vi "rsscope_core_global.vi"() -> ()   [LabVIEW 2018] (continued)
"Read Callback"="", "Write Callback"="", "Supported Models"="RTO|RTP", "Instrument Options"="", "Flags"=0, "Help"="Sets the wire on which the bus signal is measured.\n\nAvailable Repeated Capabilities:\nSerialBus: SB1, SB2, SB3, SB4\r\n\nRemote-control command(s):\nBUS<m>:ARINc:POLarity"}, {"Level"=3, "Class Only"=FALSE, "Identifier"="RSSCOPE_ATTR_PROTOCOL_ARINC429_BIT_RATE_MODE", "Descriptive Name"="Protocol ARINC429 Bit Rate Mode", "Data Type"=0, "Command"="BUS{SerialBus}:ARIN:BRM", "Access"=2, "Range Table"="rsscope_rngProtocolARINC429BitRateMode", "Read Callback"="", "Write Callback"="", "Supported Models"="RTO|RTP", "Instrument Options"="", "Flags"=0, "Help"="Sets the bit rate mode to high or low speed.\n\nAvailable Repeated Capabilities:\nSerialBus: SB1, SB2, SB3, SB4\r\n\nRemote-control command(s):\nBUS<m>:ARINc:BRMode"}, {"Level"=3, "Class Only"=FALSE, "Identifier"="RSSCOPE_ATTR_PROTOCOL_ARINC429_BIT_RATE", "Descriptive Name"="Protocol ARINC429 Bit Rate", "Data Type"=0, "Command"="BUS{SerialBus}:ARIN:BRV", "Access"=2, "Range Table"="rsscope_rngProtocolARINC429BitRate", "Read Callback"="", "Write Callback"="", "Supported Models"="RTO|RTP", "Instrument Options"="", "Flags"=0, "Help"="Sets the number of transmitted bits per second.\n\nAvailable Repeated Capabilities:\nSerialBus: SB1, SB2, SB3, SB4\r\n\nRemote-control command(s):\nBUS<m>:ARINc:BRValue"}, {"Level"=3, "Class Only"=FALSE, "Identifier"="RSSCOPE_ATTR_PROTOCOL_ARINC429_THRESHOLD_HIGH", "Descriptive Name"="Protocol ARINC429 Threshold High", "Data Type"=1, "Command"="BUS{SerialBus}:ARIN:THR:HIGH", "Access"=2, "Range Table"="rsscope_rngProtocolARINC429ThresholdHigh", "Read Callback"="", "Write Callback"="", "Supported Models"="RTO|RTP", "Instrument Options"="", "Flags"=0, "Help"="Sets the high threshold level of the signal.\n\nAvailable Repeated Capabilities:\nSerialBus: SB1, SB2, SB3, SB4\r\n\nRemote-control command(s):\nBUS<m>:ARINc:THReshold:HIGH"}, {"Level"=3, "Class Only"=FALSE, "Identifier"="RSSCOPE_ATTR_PROTOCOL_ARINC429_THRESHOLD_LOW", "Descriptive Name"="Protocol ARINC429 Threshold Low", "Data Type"=1, "Command"="BUS{SerialBus}:ARIN:THR:LOW", "Access"=2, "Range Table"="rsscope_rngProtocolARINC429ThresholdLow", "Read Callback"="", "Write Callback"="", "Supported Models"="RTO|RTP", "Instrument Options"="", "Flags"=0, "Help"="Sets the low threshold level of the signal.\n\nAvailable Repeated Capabilities:\nSerialBus: SB1, SB2, SB3, SB4\r\n\nRemote-control command(s):\nBUS<m>:ARINc:THReshold:LOW"}, {"Level"=3, "Class Only"=FALSE, "Identifier"="RSSCOPE_ATTR_PROTOCOL_ARINC429_THRESHOLD_PRESET", "Descriptive Name"="Protocol ARINC429 Threshold Preset", "Data Type"=0, "Command"="BUS{SerialBus}:ARIN:PRES", "Access"=2, "Range Table"="rsscope_rngProtocolARINC429ThresholdPreset", "Read Callback"="", "Write Callback"="", "Supported Models"="RTO|RTP", "Instrument Options"="", "Flags"=0, "Help"="Sets the default threshold voltage.\n\nAvailable Repeated Capabilities:\nSerialBus: SB1, SB2, SB3, SB4\r\n\nRemote-control command(s):\nBUS<m>:ARINc:PRESet"}, {"Level"=3, "Class Only"=TRUE, "Identifier"="", "Descriptive Name"="Timing", "Data Type"=0, "Command"="", "Access"=0, "Range Table"="", "Read Callback"="", "Write Callback"="", "Supported Models"="", "Instrument Options"="", "Flags"=0, "Help"="Specifies the ranges of the timeouts."}, {"Level"=4, "Class Only"=FALSE, "Identifier"="RSSCOPE_ATTR_PROTOCOL_ARINC429_MIN_GAP_ENABLED", "Descriptive Name"="Protocol ARINC429 Min Gap Enabled", "Data Type"=3, "Command"="BUS{SerialBus}:ARIN:MING:SEL", "Access"=2, "Range Table"="", "Read Callback"="", "Write Callback"="", "Supported Models"="RTO|RTP", "Instrument Options"="", "Flags"=0, "Help"="Enables the selection of the min gap.\n\nAvailable Repeated Capabilities:\nSerialBus: SB1, SB2, SB3, SB4\r\n\nRemote-control command(s):\nBUS<m>:ARINc:MINGap:SELect"}, {"Level"=4, "Class Only"=FALSE, "Identifier"="RSSCOPE_ATTR_PROTOCOL_ARINC429_MIN_GAP_BITS", "Descriptive Name"="Protocol ARINC429 Min Gap Bits", "Data Type"=0, "Command"="BUS{SerialBus}:ARIN:MING:BITS", "Access"=2, "Range Table"="rsscope_rngProtocolARINC429MinGapBits", "Read Callback"="", "Write Callback"="", "Supported Models"="RTO|RTP", "Instrument Options"="", "Flags"=0, "Help"="Sets a value for the min timing gap between two words.\n\nAvailable Repeated Capabilities:\nSerialBus: SB1, SB2, SB3, SB4\r\n\nRemote-control command(s):\nBUS<m>:ARINc:MINGap:BITS"}, {"Level"=4, "Class Only"=FALSE, "Identifier"="RSSCOPE_ATTR_PROTOCOL_ARINC429_MAX_GAP_ENABLED", "Descriptive Name"="Protocol ARINC429 Max Gap Enabled", "Data Type"=3, "Command"="BUS{SerialBus}:ARIN:MAXG:SEL", "Access"=2, "Range Table"="", "Read Callback"="", "Write Callback"="", "Supported Models"="RTO|RTP", "Instrument Options"="", "Flags"=0, "Help"="Enables the selection of the max gap.\n\nAvailable Repeated Capabilities:\nSerialBus: SB1, SB2, SB3, SB4\r\n\nRemote-control command(s):\nBUS<m>:ARINc:MAXGap:SELect"}, {"Level"=4, "Class Only"=FALSE, "Identifier"="RSSCOPE_ATTR_PROTOCOL_ARINC429_MAX_GAP_BITS", "Descriptive Name"="Protocol ARINC429 Max Gap Bits", "Data Type"=0, "Command"="BUS{SerialBus}:ARIN:MAXG:BITS", "Access"=2, "Range Table"="rsscope_rngProtocolARINC429MaxGapBits", "Read Callback"="", "Write Callback"="", "Supported Models"="RTO|RTP", "Instrument Options"="", "Flags"=0, "Help"="Sets the value for the maximum response time.\n\nAvailable Repeated Capabilities:\nSerialBus: SB1, SB2, SB3, SB4\r\n\nRemote-control command(s):\nBUS<m>:ARINc:MAXGap:BITS"}, {"Level"=3, "Class Only"=TRUE, "Identifier"="", "Descriptive Name"="Decoding Results", "Data Type"=0, "Command"="", "Access"=0, "Range Table"="", "Read Callback"="", "Write Callback"="", "Supported Models"="", "Instrument Options"="", "Flags"=0, "Help"="Returns the decoding result of the specified word."}, {"Level"=4, "Class Only"=FALSE, "Identifier"="RSSCOPE_ATTR_PROTOCOL_ARINC429_DECODING_RESULTS_WORDS_COUNT", "Descriptive Name"="Protocol ARINC429 Decoding Results Words Count", "Data Type"=0, "Command"="BUS{SerialBus}:ARIN:WCO?", "Access"=0, "Range Table"="", "Read Callback"="", "Write Callback"="", "Supported Models"="RTO|RTP", "Instrument Options"="", "Flags"=0, "Help"="Returns the number of decoded words.\n\nAvailable Repeated Capabilities:\nSerialBus: SB1, SB2, SB3, SB4\r\n\nRemote-control command(s):\nBUS<m>:ARINc:WCOunt?"}, {"Level"=2, "Class Only"=TRUE, "Identifier"="", "Descriptive Name"="RFFE", "Data Type"=0, "Command"="", "Access"=0, "Range Table"="", "Read Callback"="", "Write Callback"="", "Supported Models"="", "Instrument Options"="", "Flags"=0, "Help"="This class contains attributes that configure the RFFE (Radio Frequency Front-End)\n\nAttributes in this class require option R&S RTO-K40."}, {"Level"=3, "Class Only"=FALSE, "Identifier"="RSSCOPE_ATTR_PROTOCOL_RFFE_CLOCK_SOURCE", "Descriptive Name"="Protocol RFFE Clock Source", "Data Type"=0, "Command"="BUS{SerialBus}:RFFE:CLOC:SOUR", "Access"=2, "Range Table"="rsscope_rngProtocolWaveformSource", "Read Callback"="", "Write Callback"="", "Supported Models"="", "Instrument Options"="K40", "Flags"=0, "Help"="Sets the source of the RFFE clock line.\n\nAvailable Repeated Capabilities:\nSerialBus: SB1, SB2, SB3, SB4\r\n\nRemote-control command(s):\nBUS<m>:RFFE:CLOCk:SOURce"}, {"Level"=3, "Class Only"=FALSE, "Identifier"="RSSCOPE_ATTR_PROTOCOL_RFFE_DATA_SOURCE", "Descriptive Name"="Protocol RFFE Data Source", "Data Type"=0, "Command"="BUS{SerialBus}:RFFE:DATA:SOUR", "Access"=2, "Range Table"="rsscope_rngProtocolWaveformSource", "Read Callback"="", "Write Callback"="", "Supported Models"="", "Instrument Options"="K40", "Flags"=0, "Help"="Sets the source of the RFFE data line.\n\nAvailable Repeated Capabilities:\nSerialBus: SB1, SB2, SB3, SB4\r\n\nRemote-control command(s):\nBUS<m>:RFFE:DATA:SOURce"}, {"Level"=3, "Class Only"=FALSE, "Identifier"="RSSCOPE_ATTR_PROTOCOL_RFFE_PRESET_THRESHOLD", "Descriptive Name"="Protocol RFFE Preset Threshold", "Data Type"=0, "Command"="BUS{SerialBus}:RFFE:PRES", "Access"=2, "Range Table"="rsscope_rngProtocolRFFEPreset", "Read Callback"="", "Write Callback"="", "Supported Models"="", "Instrument Options"="K40", "Flags"=0, "Help"="Sets default threshold voltages for 1.2 V or 1.8 V bus. Set the value to Manual if you want to define individual thresholds.\n\nAvailable Repeated Capabilities:\nSerialBus: SB1, SB2, SB3, SB4\r\n\nRemote-control command(s):\nBUS<m>:RFFE:PRESet"}, {"Level"=3, "Class Only"=FALSE, "Identifier"="RSSCOPE_ATTR_PROTOCOL_RFFE_CLOCK_THRESHOLD_HIGH", "Descriptive Name"="Protocol RFFE Clock Threshold High", "Data Type"=1, "Command"="BUS{SerialBus}:RFFE:CLOC:THR:HIGH", "Access"=2, "Range Table"="RsScope_rngProtocolRFFEThreshold", "Read Callback"="", "Write Callback"="", "Supported Models"="", "Instrument Options"="K40", "Flags"=0, "Help"="Set the positive going thresholds.\n\nAvailable Repeated Capabilities:\nSerialBus: SB1, SB2, SB3, SB4\r\n\nRemote-control command(s):\nBUS<m>:RFFE:CLOCk:THReshold:HIGH"}, {"Level"=3, "Class Only"=FALSE, "Identifier"="RSSCOPE_ATTR_PROTOCOL_RFFE_CLOCK_THRESHOLD_LOW", "Descriptive Name"="Protocol RFFE Clock Threshold Low", "Data Type"=1, "Command"="BUS{SerialBus}:RFFE:CLOC:THR:LOW", "Access"=2, "Range Table"="RsScope_rngProtocolRFFEThreshold", "Read Callback"="", "Write Callback"="", "Supported Models"="", "Instrument Options"="K40", "Flags"=0, "Help"="Sets the negative going thresholds.\n\nAvailable Repeated Capabilities:\nSerialBus: SB1, SB2, SB3, SB4\r\n\nRemote-control command(s):\nBUS<m>:RFFE:CLOCk:THReshold:LOW"}, {"Level"=3, "Class Only"=FALSE, "Identifier"="RSSCOPE_ATTR_PROTOCOL_RFFE_CLOCK_THRESHOLD_HYSTERESIS", "Descriptive Name"="Protocol RFFE Clock Threshold Hysteresis", "Data Type"=1, "Command"="BUS{SerialBus}:RFFE:CLOC:THR:HYST", "Access"=2, "Range Table"="rsscope_rngProtocolRFFEThresholdHysteresis", "Read Callback"="", "Write Callback"="", "Supported Models"="", "Instrument Options"="K40", "Flags"=0, "Help"="Sets the hysteresises between V TP  and V TN.\n\nAvailable Repeated Capabilities:\nSerialBus: SB1, SB2, SB3, SB4\r\n\nRemote-control command(s):\nBUS<m>:RFFE:CLOCk:THReshold:HYSTeresis"}, {"Level"=3, "Class Only"=FALSE, "Identifier"="RSSCOPE_ATTR_PROTOCOL_RFFE_DATA_THRESHOLD_HIGH", "Descriptive Name"="Protocol RFFE Data Threshold High", "Data Type"=1, "Command"="BUS{SerialBus}:RFFE:DATA:THR:HIGH", "Access"=2, "Range Table"="RsScope_rngProtocolRFFEThreshold", "Read Callback"="", "Write Callback"="", "Supported Models"="", "Instrument Options"="K40", "Flags"=0, "Help"="Set the positive going thresholds.\n\nAvailable Repeated Capabilities:\nSerialBus: SB1, SB2, SB3, SB4\r\n\nRemote-control command(s):\nBUS<m>:RFFE:DATA:THReshold:HIGH"}, {"Level"=3, "Class Only"=FALSE, "Identifier"="RSSCOPE_ATTR_PROTOCOL_RFFE_DATA_THRESHOLD_LOW", "Descriptive Name"="Protocol RFFE Data Threshold Low", "Data Type"=1, "Command"="BUS{SerialBus}:RFFE:DATA:THR:LOW", "Access"=2, "Range Table"="RsScope_rngProtocolRFFEThreshold", "Read Callback"="", "Write Callback"="", "Supported Models"="", "Instrument Options"="K40", "Flags"=0, "Help"="Sets the negative going thresholds.\n\nAvailable Repeated Capabilities:\nSerialBus: SB1, SB2, SB3, SB4\r\n\nRemote-control command(s):\nBUS<m>:RFFE:DATA:THReshold:LOW"}, {"Level"=3, "Class Only"=FALSE, "Identifier"="RSSCOPE_ATTR_PROTOCOL_RFFE_DATA_THRESHOLD_HYSTERESIS", "Descriptive Name"="Protocol RFFE Data Threshold Hysteresis", "Data Type"=1, "Command"="BUS{SerialBus}:RFFE:DATA:THR:HYST", "Access"=2, "Range Table"="rsscope_rngProtocolRFFEThresholdHysteresis", "Read Callback"="", "Write Callback"="", "Supported Models"="", "Instrument Options"="K40", "Flags"=0, "Help"="Sets the hysteresises between V TP  and V TN.\n\nAvailable Repeated Capabilities:\nSerialBus: SB1, SB2, SB3, SB4\r\n\nRemote-control command(s):\nBUS<m>:RFFE:DATA:THReshold:HYSTeresis"}, {"Level"=3, "Class Only"=FALSE, "Identifier"="RSSCOPE_ATTR_PROTOCOL_RFFE_THRESHOLDS_COUPLING", "Descriptive Name"="Protocol RFFE Thresholds Coupling", "Data Type"=3, "Command"="BUS{SerialBus}:RFFE:COUP", "Access"=2, "Range Table"="", "Read Callback"="", "Write Callback"="", "Supported Models"="", "Instrument Options"="K40", "Flags"=0, "Help"="If enabled, the data line thresholds are set to the clock line threshold values.\n\nAvailable Repeated Capabilities:\nSerialBus: SB1, SB2, SB3, SB4\r\n\nRemote-control command(s):\nBUS<m>:RFFE:COUPling"}, {"Level"=3, "Class Only"=FALSE, "Identifier"="RSSCOPE_ATTR_PROTOCOL_RFFE_GLITCH_FILTER_ENABLED", "Descriptive Name"="Protocol RFFE Glitch Filter Enabled", "Data Type"=3, "Command"="BUS{SerialBus}:RFFE:GFIL", "Access"=2, "Range Table"="", "Read Callback"="", "Write Callback"="", "Supported Models"="", "Instrument Options"="K40", "Flags"=0, "Help"="Enables the glitch filter on the clock and data lines to improve decode accuracy.\n\nAvailable Repeated Capabilities:\nSerialBus: SB1, SB2, SB3, SB4\r\n\nRemote-control command(s):\nBUS<m>:RFFE:GFILter"}, {"Level"=3, "Class Only"=FALSE, "Identifier"="RSSCOPE_ATTR_PROTOCOL_RFFE_GLITCH_FILTER_WIDTH", "Descriptive Name"="Protocol RFFE Glitch Filter Width", "Data Type"=1, "Command"="BUS{SerialBus}:RFFE:GFW", "Access"=2, "Range Table"="rsscope_rngProtocolRFFEGlitchFilterWidth", "Read Callback"="", "Write Callback"="", "Supported Models"="", "Instrument Options"="K40", "Flags"=0, "Help"="Sets the maximum glitch width to be ignored\n\nAvailable Repeated Capabilities:\nSerialBus: SB1, SB2, SB3, SB4\r\n\nRemote-control command(s):\nBUS<m>:RFFE:GFWidth"}, {"Level"=3, "Class Only"=FALSE, "Identifier"="RSSCOPE_ATTR_PROTOCOL_RFFE_MIN_GAP_ENABLED", "Descriptive Name"="Protocol RFFE Min Gap Enabled", "Data Type"=3, "Command"="BUS{SerialBus}:RFFE:MING:SEL", "Access"=2, "Range Table"="", "Read Callback"="", "Write Callback"="", "Supported Models"="", "Instrument Options"="K40", "Flags"=0, "Help"="Enables the selection of the min gap.\n\nAvailable Repeated Capabilities:\nSerialBus: SB1, SB2, SB3, SB4\r\n\nRemote-control command(s):\nBUS<m>:RFFE:MINGap:SELect"}, {"Level"=3, "Class Only"=FALSE, "Identifier"="RSSCOPE_ATTR_PROTOCOL_RFFE_MIN_GAP_TIME", "Descriptive Name"="Protocol RFFE Min Gap Time", "Data Type"=1, "Command"="BUS{SerialBus}:RFFE:MING:TIME", "Access"=2, "Range Table"="rsscope_rngProtocolRFFEMinGapTime", "Read Callback"="", "Write Callback"="", "Supported Models"="", "Instrument Options"="K40", "Flags"=0, "Help"="Sets the minimum idle time between the Bus Park Cycle (BP) and Sequence Start Condition (SSC).\n\nAvailable Repeated Capabilities:\nSerialBus: SB1, SB2, SB3, SB4\r\n\nRemote-control command(s):\nBUS<m>:RFFE:MINGap:TIME"}, {"Level"=3, "Class Only"=FALSE, "Identifier"="RSSCOPE_ATTR_PROTOCOL_RFFE_MAX_GAP_ENABLED", "Descriptive Name"="Protocol RFFE Max Gap Enabled", "Data Type"=3, "Command"="BUS{SerialBus}:RFFE:MAXG:SEL", "Access"=2, "Range Table"="", "Read Callback"="", "Write Callback"="", "Supported Models"="", "Instrument Options"="K40", "Flags"=0, "Help"="Enables the selection of the max gap.\n\nAvailable Repeated Capabilities:\nSerialBus: SB1, SB2, SB3, SB4\r\n\nRemote-control command(s):\nBUS<m>:RFFE:MAXGap:SELect"}, {"Level"=3, "Class Only"=FALSE, "Identifier"="RSSCOPE_ATTR_PROTOCOL_RFFE_MAX_GAP_TIME", "Descriptive Name"="Protocol RFFE Max Gap Time", "Data Type"=1, "Command"="BUS{SerialBus}:RFFE:MAXG:TIME", "Access"=2, "Range Table"="RsScope_rngProtocolRFFEMaxGapTime", "Read Callback"="", "Write Callback"="", "Supported Models"="", "Instrument Options"="K40", "Flags"=0, "Help"="Sets the maximum idle time between the Bus Park Cycle (BP) and Sequence Start Condition (SSC).\n\nAvailable Repeated Capabilities:\nSerialBus: SB1, SB2, SB3, SB4\r\n\nRemote-control command(s):\nBUS<m>:RFFE:MAXGap:TIME"}, {"Level"=3, "Class Only"=FALSE, "Identifier"="RSSCOPE_ATTR_PROTOCOL_RFFE_READ_MODE", "Descriptive Name"="Protocol RFFE Read Mode", "Data Type"=0, "Command"="BUS{SerialBus}:RFFE:RDMD", "Access"=2, "Range Table"="RsScope_rngRFFEReadMode", "Read Callback"="", "Write Callback"="", "Supported Models"="", "Instrument Options"="K40", "Flags"=0, "Help"="Selects, if the standard or synchronous read (SREAD) mode is used.\n\nAvailable Repeated Capabilities:\nSerialBus: SB1, SB2, SB3, SB4\r\n\nRemote-control command(s):\nBUS<m>:RFFE:RDMD"}, {"Level"=3, "Class Only"=FALSE, "Identifier"="RSSCOPE_ATTR_PROTOCOL_RFFE_VERSION", "Descriptive Name"="Protocol RFFE Version", "Data Type"=0, "Command"="BUS{SerialBus}:RFFE:VERS", "Access"=2, "Range Table"="RsScope_rngRFFEVersion", "Read Callback"="", "Write Callback"="", "Supported Models"="", "Instrument Options"="K40", "Flags"=0, "Help"="Selects the RFFE version.\n\nAvailable Repeated Capabilities:\nSerialBus: SB1, SB2, SB3, SB4\r\n\nRemote-control command(s):\nBUS<m>:RFFE:VERSion"}, {"Level"=3, "Class Only"=TRUE, "Identifier"="", "Descriptive Name"="Decoding Results", "Data Type"=0, "Command"="", "Access"=0, "Range Table"="", "Read Callback"="", "Write Callback"="", "Supported Models"="", "Instrument Options"="", "Flags"=0, "Help"="Returns the decoding result of the specified sequence."}, {"Level"=4, "Class Only"=FALSE, "Identifier"="RSSCOPE_ATTR_PROTOCOL_RFFE_DECODING_RESULTS_SEQUENCE_COUNT", "Descriptive Name"="Protocol RFFE Decoding Results Sequence Count", "Data Type"=0, "Command"="BUS{SerialBus}:RFFE:FCO?", "Access"=0, "Range Table"="", "Read Callback"="", "Write Callback"="", "Supported Models"="RTO|RTP", "Instrument Options"="", "Flags"=0, "Help"="Returns the number of command sequences in the current acquisition.\n\nAvailable Repeated Capabilities:\nSerialBus: SB1, SB2, SB3, SB4\r\n\nRemote-control command(s):\nBUS<m>:RFFE:FCOunt?"}, {"Level"=2, "Class Only"=TRUE, "Identifier"="", "Descriptive Name"="MDIO", "Data Type"=0, "Command"="", "Access"=0, "Range Table"="", "Read Callback"="", "Write Callback"="", "Supported Models"="", "Instrument Options"="", "Flags"=0, "Help"="This class contains attributes that configure the MDIO (Manage-\nment Data Input/Output)\n\nFunctions in this class requires option R&S RTO-K55."}, {"Level"=3, "Class Only"=FALSE, "Identifier"="RSSCOPE_ATTR_PROTOCOL_MDIO_THRESHOLD_PRESET", "Descriptive Name"="Protocol MDIO Threshold Preset", "Data Type"=0, "Command"="BUS{SerialBus}:MDIO:PRES", "Access"=2, "Range Table"="rsscope_rngProtocolMDIOThresholdPreset", "Read Callback"="", "Write Callback"="", "Supported Models"="", "Instrument Options"="K55", "Flags"=0, "Help"="Selects the default threshold settings according to the Ethernet standard.\n\nAvailable Repeated Capabilities:\nSerialBus: SB1, SB2, SB3, SB4\r\n\nRemote-control command(s):\nBUS<m>:MDIO:PRESet"}, {"Level"=3, "Class Only"=FALSE, "Identifier"="RSSCOPE_ATTR_PROTOCOL_MDIO_CLOCK_SOURCE", "Descriptive Name"="Protocol MDIO Clock Source", "Data Type"=0, "Command"="BUS{SerialBus}:MDIO:CLOC:SOUR", "Access"=2, "Range Table"="rsscope_rngProtocolWaveformSource", "Read Callback"="", "Write Callback"="", "Supported Models"="", "Instrument Options"="K55", "Flags"=0, "Help"="Selects the source for the clock line (management data clock, MDC). Permitted selections are the analog channels &apos;C1&apos;  &apos;C4&apos; and the digital channels &apos;D0&apos;  &apos;D15&apos;.\n\nAvailable Repeated Capabilities:\nSerialBus: SB1, SB2, SB3, SB4\r\n\nRemote-control command(s):\nBUS<m>:MDIO:CLOCk:SOURce"}, {"Level"=3, "Class Only"=FALSE, "Identifier"="RSSCOPE_ATTR_PROTOCOL_MDIO_CLOCK_THRESHOLD_HIGH", "Descriptive Name"="Protocol MDIO Clock Threshold High", "Data Type"=1, "Command"="BUS{SerialBus}:MDIO:CLOC:THR:HIGH", "Access"=2, "Range Table"="rsscope_rngProtocolMDIOThreshold", "Read Callback"="", "Write Callback"="", "Supported Models"="", "Instrument Options"="K55", "Flags"=0, "Help"="Defines the upper threshold level for the clock signal.\n\nAvailable Repeated Capabilities:\nSerialBus: SB1, SB2, SB3, SB4\r\n\nRemote-control command(s):\nBUS<m>:MDIO:CLOCk:THReshold:HIGH"}, {"Level"=3, "Class Only"=FALSE, "Identifier"="RSSCOPE_ATTR_PROTOCOL_MDIO_CLOCK_THRESHOLD_LOW", "Descriptive Name"="Protocol MDIO Clock Threshold Low", "Data Type"=1, "Command"="BUS{SerialBus}:MDIO:CLOC:THR:LOW", "Access"=2, "Range Table"="rsscope_rngProtocolMDIOThreshold", "Read Callback"="", "Write Callback"="", "Supported Models"="", "Instrument Options"="K55", "Flags"=0, "Help"="Defines the lower threshold level for the clock signal.\n\nAvailable Repeated Capabilities:\nSerialBus: SB1, SB2, SB3, SB4\r\n\nRemote-control command(s):\nBUS<m>:MDIO:CLOCk:THReshold:LOW"}, {"Level"=3, "Class Only"=FALSE, "Identifier"="RSSCOPE_ATTR_PROTOCOL_MDIO_DATA_SOURCE", "Descriptive Name"="Protocol MDIO Data Source", "Data Type"=0, "Command"="BUS{SerialBus}:MDIO:DATA:SOUR", "Access"=2, "Range Table"="rsscope_rngProtocolWaveformSource", "Read Callback"="", "Write Callback"="", "Supported Models"="", "Instrument Options"="K55", "Flags"=0, "Help"="Selects the source for the data signal. Permitted selections are the analog channels &apos;C1&apos;  &apos;C4&apos; and the digital channels &apos;D0&apos;  &apos;D15&apos;.\n\nAvailable Repeated Capabilities:\nSerialBus: SB1, SB2, SB3, SB4\r\n\nRemote-control command(s):\nBUS<m>:MDIO:DATA:SOURce"}, {"Level"=3, "Class Only"=FALSE, "Identifier"="RSSCOPE_ATTR_PROTOCOL_MDIO_DATA_THRESHOLD_HIGH", "Descriptive Name"="Protocol MDIO Data Threshold High", "Data Type"=1, "Command"="BUS{SerialBus}:MDIO:DATA:THR:HIGH", "Access"=2, "Range Table"="rsscope_rngProtocolMDIOThreshold", "Read Callback"="", "Write Callback"="", "Supported Models"="", "Instrument Options"="K55", "Flags"=0, "Help"="Defines the upper threshold level for the data signal.\n\nAvailable Repeated Capabilities:\nSerialBus: SB1, SB2, SB3, SB4\r\n\nRemote-control command(s):\nBUS<m>:MDIO:DATA:THReshold:HIGH"}, {"Level"=3, "Class Only"=FALSE, "Identifier"="RSSCOPE_ATTR_PROTOCOL_MDIO_DATA_THRESHOLD_LOW", "Descriptive Name"="Protocol MDIO Data Threshold Low", "Data Type"=1, "Command"="BUS{SerialBus}:MDIO:DATA:THR:LOW", "Access"=2, "Range Table"="rsscope_rngProtocolMDIOThreshold", "Read Callback"="", "Write Callback"="", "Supported Models"="", "Instrument Options"="K55", "Flags"=0, "Help"="Defines the lower threshold level for the data signal.\n\nAvailable Repeated Capabilities:\nSerialBus: SB1, SB2, SB3, SB4\r\n\nRemote-control command(s):\nBUS<m>:MDIO:DATA:THReshold:LOW"}, {"Level"=3, "Class Only"=FALSE, "Identifier"="RSSCOPE_ATTR_PROTOCOL_MDIO_THRESHOLDS_COUPLING", "Descriptive Name"="Protocol MDIO Thresholds Coupling", "Data Type"=3, "Command"="BUS{SerialBus}:MDIO:COUP", "Access"=2, "Range Table"="", "Read Callback"="", "Write Callback"="", "Supported Models"="", "Instrument Options"="K55", "Flags"=0, "Help"="If enabled, the data line thresholds are set to the clock line threshold values.\n\nAvailable Repeated Capabilities:\nSerialBus: SB1, SB2, SB3, SB4\r\n\nRemote-control command(s):\nBUS<m>:MDIO:COUPling"}, {"Level"=3, "Class Only"=FALSE, "Identifier"="RSSCOPE_ATTR_PROTOCOL_MDIO_MAX_GAP_TIME", "Descriptive Name"="Protocol MDIO Max Gap Time", "Data Type"=1, "Command"="BUS{SerialBus}:MDIO:MAXG", "Access"=2, "Range Table"="RsScope_rngMDIOMaxGapTime", "Read Callback"="", "Write Callback"="", "Supported Models"="", "Instrument Options"="", "Flags"=0, "Help"="Sets the maximum idle time between two frames.\n\nAvailable Repeated Capabilities:\nSerialBus: SB1, SB2, SB3, SB4\r\n\nRemote-control command(s):\nBUS<m>:MDIO:MAXGap"}, {"Level"=3, "Class Only"=TRUE, "Identifier"="", "Descriptive Name"="Decoding Results", "Data Type"=0, "Command"="", "Access"=0, "Range Table"="", "Read Callback"="", "Write Callback"="", "Supported Models"="", "Instrument Options"="", "Flags"=0, "Help"="Returns the decoding result of the specified word."}, {"Level"=4, "Class Only"=FALSE, "Identifier"="RSSCOPE_ATTR_PROTOCOL_MDIO_DECODING_RESULTS_WORD_COUNT", "Descriptive Name"="Protocol MDIO Decoding Results Word Count", "Data Type"=0, "Command"="BUS{SerialBus}:MDIO:WCO?", "Access"=0, "Range Table"="", "Read Callback"="", "Write Callback"="", "Supported Models"="", "Instrument Options"="K55", "Flags"=0, "Help"="Returns the number of decoded words.\n\nAvailable Repeated Capabilities:\nSerialBus: SB1, SB2, SB3, SB4\r\n\nRemote-control command(s):\nBUS<m>:MDIO:WCOunt?"}, {"Level"=2, "Class Only"=TRUE, "Identifier"="", "Descriptive Name"="Ethernet", "Data Type"=0, "Command"="", "Access"=0, "Range Table"="", "Read Callback"="", "Write Callback"="", "Supported Models"="", "Instrument Options"="", "Flags"=0, "Help"="This class contains attributes that configure the  Ethernet protocol variants 10BASE-T and 100BASE-TX.\n\nAttributes in this class require option R&S RTO-K8."}, {"Level"=3, "Class Only"=FALSE, "Identifier"="RSSCOPE_ATTR_PROTOCOL_ETHERNET_VARIANT", "Descriptive Name"="Protocol Ethernet Variant", "Data Type"=0, "Command"="BUS{SerialBus}:ETH:VAR", "Access"=2, "Range Table"="rsscope_rngProtocolEthernetVariant", "Read Callback"="", "Write Callback"="", "Supported Models"="", "Instrument Options"="K8", "Flags"=0, "Help"="Selects the Ethernet protocol variant and transmission speed.\n\nAvailable Repeated Capabilities:\nSerialBus: SB1, SB2, SB3, SB4\r\n\nRemote-control command(s):\nBUS<m>:ETHernet:VARiant"}, {"Level"=3, "Class Only"=FALSE, "Identifier"="RSSCOPE_ATTR_PROTOCOL_ETHERNET_SOURCE", "Descriptive Name"="Protocol Ethernet Source", "Data Type"=0, "Command"="BUS{SerialBus}:ETH:SOUR", "Access"=2, "Range Table"="rsscope_rngProtocolWaveformSource", "Read Callback"="", "Write Callback"="", "Supported Models"="", "Instrument Options"="K8", "Flags"=0, "Help"="Selects the source channel for the data signal. Usually, the source is one of the analog channels. Reference and math waveforms are available as source if the trigger source is one of the analog channels but not the serial\nbus.\n\nAvailable Repeated Capabilities:\nSerialBus: SB1, SB2, SB3, SB4\r\n\nRemote-control command(s):\nBUS<m>:ETHernet:SOURce"}, {"Level"=3, "Class Only"=FALSE, "Identifier"="RSSCOPE_ATTR_PROTOCOL_ETHERNET_POLARITY", "Descriptive Name"="Protocol Ethernet Polarity", "Data Type"=0, "Command"="BUS{SerialBus}:ETH:POL", "Access"=2, "Range Table"="rsscope_rngEthernetPolarity", "Read Callback"="", "Write Callback"="", "Supported Models"="", "Instrument Options"="K8", "Flags"=0, "Help"="Defines the polarity of the data signal. This setting is only available in 10BASE-T.\n\nAvailable Repeated Capabilities:\nSerialBus: SB1, SB2, SB3, SB4\r\n\nRemote-control command(s):\nBUS<m>:ETHernet:POLarity"}, {"Level"=3, "Class Only"=FALSE, "Identifier"="RSSCOPE_ATTR_PROTOCOL_ETHERNET_THRESHOLD_PRESET", "Descriptive Name"="Protocol Ethernet Threshold Preset", "Data Type"=0, "Command"="BUS{SerialBus}:ETH:PRES", "Access"=2, "Range Table"="rsscope_rngProtocolEthernetThresholdPreset", "Read Callback"="", "Write Callback"="", "Supported Models"="", "Instrument Options"="K8", "Flags"=0, "Help"="Sets the thresholds to predefined or individually definable voltage levels.\n\nAvailable Repeated Capabilities:\nSerialBus: SB1, SB2, SB3, SB4\r\n\nRemote-control command(s):\nBUS<m>:ETHernet:PRESet"}, {"Level"=3, "Class Only"=FALSE, "Identifier"="RSSCOPE_ATTR_PROTOCOL_ETHERNET_THRESHOLD_LOW", "Descriptive Name"="Protocol Ethernet Threshold Low", "Data Type"=1, "Command"="BUS{SerialBus}:ETH:THR:LOW", "Access"=2, "Range Table"="rsscope_rngProtocolEthernetThresholdLow", "Read Callback"="", "Write Callback"="", "Supported Models"="", "Instrument Options"="K8", "Flags"=0, "Help"="Sets the lower threshold value for the signal digitization. If the signal value is below this threshold, the signal state is considered low.\n\nAvailable Repeated Capabilities:\nSerialBus: SB1, SB2, SB3, SB4\r\n\nRemote-control command(s):\nBUS<m>:ETHernet:THReshold:LOW"}, {"Level"=3, "Class Only"=FALSE, "Identifier"="RSSCOPE_ATTR_PROTOCOL_ETHERNET_THRESHOLD_HIGH", "Descriptive Name"="Protocol Ethernet Threshold High", "Data Type"=1, "Command"="BUS{SerialBus}:ETH:THR:HIGH", "Access"=2, "Range Table"="rsscope_rngProtocolEthernetThresholdHigh", "Read Callback"="", "Write Callback"="", "Supported Models"="", "Instrument Options"="K8", "Flags"=0, "Help"="Sets the upper threshold value for the signal digitization. If the signal value is higher than the this threshold, the signal state is considered high.\n\nAvailable Repeated Capabilities:\nSerialBus: SB1, SB2, SB3, SB4\r\n\nRemote-control command(s):\nBUS<m>:ETHernet:THReshold:HIGH"}, {"Level"=3, "Class Only"=FALSE, "Identifier"="RSSCOPE_ATTR_PROTOCOL_ETHERNET_BIT_RATE", "Descriptive Name"="Protocol Ethernet Bit Rate", "Data Type"=0, "Command"="BUS{SerialBus}:ETH:BITR", "Access"=2, "Range Table"="rsscope_rngProtocolEthernetBitRate", "Read Callback"="", "Write Callback"="", "Supported Models"="", "Instrument Options"="K8", "Flags"=0, "Help"="Sets the bit rate value that defines the transmission speed in bits per second.\n\nAvailable Repeated Capabilities:\nSerialBus: SB1, SB2, SB3, SB4\r\n\nRemote-control command(s):\nBUS<m>:ETHernet:BITRate"}, {"Level"=3, "Class Only"=TRUE, "Identifier"="", "Descriptive Name"="Decoding Results", "Data Type"=0, "Command"="", "Access"=0, "Range Table"="", "Read Callback"="", "Write Callback"="", "Supported Models"="", "Instrument Options"="", "Flags"=0, "Help"="Returns the decoding result of the specified word."}, {"Level"=4, "Class Only"=FALSE, "Identifier"="RSSCOPE_ATTR_PROTOCOL_ETHERNET_DECODING_RESULTS_WORD_COUNT", "Descriptive Name"="Protocol Ethernet Decoding Results Word Count", "Data Type"=0, "Command"="BUS{SerialBus}:ETH:WCO?", "Access"=0, "Range Table"="", "Read Callback"="", "Write Callback"="", "Supported Models"="", "Instrument Options"="K8", "Flags"=0, "Help"="Returns the number of decoded words.\n\nAvailable Repeated Capabilities:\nSerialBus: SB1, SB2, SB3, SB4\r\n\nRemote-control command(s):\nBUS<m>:ETHernet:WCOunt?"}, {"Level"=2, "Class Only"=TRUE, "Identifier"="", "Descriptive Name"="USB", "Data Type"=0, "Command"="", "Access"=0, "Range Table"="", "Read Callback"="", "Write Callback"="", "Supported Models"="", "Instrument Options"="", "Flags"=0, "Help"="This class contains functions that configure the USB (Universal\nSerial Bus).\n\nFunctions in this class requires option R&S RTO-K60."}, {"Level"=3, "Class Only"=FALSE, "Identifier"="RSSCOPE_ATTR_PROTOCOL_USB_D_PLUS_SOURCE", "Descriptive Name"="Protocol USB D Plus Source", "Data Type"=0, "Command"="BUS{SerialBus}:USB:DPL:SOUR", "Access"=2, "Range Table"="rsscope_rngProtocolUSBWaveformSource", "Read Callback"="", "Write Callback"="", "Supported Models"="", "Instrument Options"="K60", "Flags"=0, "Help"="Selects the source for the D+ data signal (in USB low speed and USB full speed protocol, only).\n\nAvailable Repeated Capabilities:\nSerialBus: SB1, SB2, SB3, SB4\r\n\nRemote-control command(s):\nBUS<m>:USB:DPLus:SOURce"}, {"Level"=3, "Class Only"=FALSE, "Identifier"="RSSCOPE_ATTR_PROTOCOL_USB_D_MINUS_SOURCE", "Descriptive Name"="Protocol USB D Minus Source", "Data Type"=0, "Command"="BUS{SerialBus}:USB:DMIN:SOUR", "Access"=2, "Range Table"="rsscope_rngProtocolUSBWaveformSource", "Read Callback"="", "Write Callback"="", "Supported Models"="", "Instrument Options"="K60", "Flags"=0, "Help"="Selects the source for the D- data signal (in USB low speed and USB full speed protocol, only).\n\nAvailable Repeated Capabilities:\nSerialBus: SB1, SB2, SB3, SB4\r\n\nRemote-control command(s):\nBUS<m>:USB:DMINus:SOURce"}, {"Level"=3, "Class Only"=FALSE, "Identifier"="RSSCOPE_ATTR_PROTOCOL_USB_DIFFERENTIAL_SOURCE", "Descriptive Name"="Protocol USB Differential Source", "Data Type"=0, "Command"="BUS{SerialBus}:USB:DIFF:SOUR", "Access"=2, "Range Table"="rsscope_rngProtocolUSBWaveformSource", "Read Callback"="", "Write Callback"="", "Supported Models"="", "Instrument Options"="K60", "Flags"=0, "Help"="Selects the source for the differential signal in the USB high speed protocol.\n\nAvailable Repeated Capabilities:\nSerialBus: SB1, SB2, SB3, SB4\r\n\nRemote-control command(s):\nBUS<m>:USB:DIFFerential:SOURce"}, {"Level"=3, "Class Only"=FALSE, "Identifier"="RSSCOPE_ATTR_PROTOCOL_USB_DATA_SOURCE", "Descriptive Name"="Protocol USB Data Source", "Data Type"=0, "Command"="BUS{SerialBus}:USB:DATA:SOUR", "Access"=2, "Range Table"="rsscope_rngProtocolUSBWaveformSource", "Read Callback"="", "Write Callback"="", "Supported Models"="", "Instrument Options"="K60", "Flags"=0, "Help"="Selects the source for the data signal in the USB HSIC protocol.\n\nAvailable Repeated Capabilities:\nSerialBus: SB1, SB2, SB3, SB4\r\n\nRemote-control command(s):\nBUS<m>:USB:DATA:SOURce"}, {"Level"=3, "Class Only"=FALSE, "Identifier"="RSSCOPE_ATTR_PROTOCOL_USB_STROBE_SOURCE", "Descriptive Name"="Protocol USB Strobe Source", "Data Type"=0, "Command"="BUS{SerialBus}:USB:STR:SOUR", "Access"=2, "Range Table"="rsscope_rngProtocolUSBWaveformSource", "Read Callback"="", "Write Callback"="", "Supported Models"="", "Instrument Options"="K60", "Flags"=0, "Help"="Selects the source for the strobe signal in the USB HSIC protocol.\n\nAvailable Repeated Capabilities:\nSerialBus: SB1, SB2, SB3, SB4\r\n\nRemote-control command(s):\nBUS<m>:USB:STRobe:SOURce"}, {"Level"=3, "Class Only"=FALSE, "Identifier"="RSSCOPE_ATTR_PROTOCOL_USB_TECHNOLOGY", "Descriptive Name"="Protocol USB Technology", "Data Type"=0, "Command"="BUS{SerialBus}:USB:TECH", "Access"=2, "Range Table"="rsscope_rngProtocolUSBTechnology", "Read Callback"="", "Write Callback"="", "Supported Models"="", "Instrument Options"="K60", "Flags"=0, "Help"="Defines the USB protocol technology and transmission speed.\n\nAvailable Repeated Capabilities:\nSerialBus: SB1, SB2, SB3, SB4\r\n\nRemote-control command(s):\nBUS<m>:USB:TECHnology"}, {"Level"=3, "Class Only"=FALSE, "Identifier"="RSSCOPE_ATTR_PROTOCOL_USB_D_PLUS_THRESHOLD", "Descriptive Name"="Protocol USB D Plus Threshold", "Data Type"=1, "Command"="BUS{SerialBus}:USB:DPL:THR", "Access"=2, "Range Table"="rsscope_rngProtocolUSBThreshold", "Read Callback"="", "Write Callback"="", "Supported Models"="", "Instrument Options"="K60", "Flags"=0, "Help"="Defines the threshold level for the D+ data signal (in USB low speed and USB full speed protocol, only).\n\nAvailable Repeated Capabilities:\nSerialBus: SB1, SB2, SB3, SB4\r\n\nRemote-control command(s):\nBUS<m>:USB:DPLus:THReshold"}, {"Level"=3, "Class Only"=FALSE, "Identifier"="RSSCOPE_ATTR_PROTOCOL_USB_D_MINUS_THRESHOLD", "Descriptive Name"="Protocol USB D Minus Threshold", "Data Type"=1, "Command"="BUS{SerialBus}:USB:DMIN:THR", "Access"=2, "Range Table"="rsscope_rngProtocolUSBThreshold", "Read Callback"="", "Write Callback"="", "Supported Models"="", "Instrument Options"="K60", "Flags"=0, "Help"="Defines the threshold level for the D- data signal (in USB low speed and USB full speed protocol, only).\n\nAvailable Repeated Capabilities:\nSerialBus: SB1, SB2, SB3, SB4\r\n\nRemote-control command(s):\nBUS<m>:USB:DMINus:THReshold"}, {"Level"=3, "Class Only"=FALSE, "Identifier"="RSSCOPE_ATTR_PROTOCOL_USB_DIFFERENTIAL_THRESHOLD", "Descriptive Name"="Protocol USB Differential Threshold", "Data Type"=1, "Command"="BUS{SerialBus}:USB:DIFF:THR", "Access"=2, "Range Table"="rsscope_rngProtocolUSBThresholdHighSpeed", "Read Callback"="", "Write Callback"="", "Supported Models"="", "Instrument Options"="K60", "Flags"=0, "Help"="Defines the threshold level for the differential signal in the USB high speed protocol.\n\nAvailable Repeated Capabilities:\nSerialBus: SB1, SB2, SB3, SB4\r\n\nRemote-control command(s):\nBUS<m>:USB:DIFFerential:THReshold"}, {"Level"=3, "Class Only"=FALSE, "Identifier"="RSSCOPE_ATTR_PROTOCOL_USB_DATA_THRESHOLD", "Descriptive Name"="Protocol USB Data Threshold", "Data Type"=1, "Command"="BUS{SerialBus}:USB:DATA:THR", "Access"=2, "Range Table"="rsscope_rngProtocolUSBThresholdHighSpeed", "Read Callback"="", "Write Callback"="", "Supported Models"="", "Instrument Options"="K60", "Flags"=0, "Help"="Defines the threshold level for the data signal in the USB HSIC protocol.\n\nAvailable Repeated Capabilities:\nSerialBus: SB1, SB2, SB3, SB4\r\n\nRemote-control command(s):\nBUS<m>:USB:DATA:THReshold"}, {"Level"=3, "Class Only"=FALSE, "Identifier"="RSSCOPE_ATTR_PROTOCOL_USB_STROBE_THRESHOLD", "Descriptive Name"="Protocol USB Strobe Threshold", "Data Type"=1, "Command"="BUS{SerialBus}:USB:STR:THR", "Access"=2, "Range Table"="rsscope_rngProtocolUSBThresholdHighSpeed", "Read Callback"="", "Write Callback"="", "Supported Models"="", "Instrument Options"="K60", "Flags"=0, "Help"="Defines the threshold level for the strobe signal in the USB HSIC protocol.\n\nAvailable Repeated Capabilities:\nSerialBus: SB1, SB2, SB3, SB4\r\n\nRemote-control command(s):\nBUS<m>:USB:STRobe:THReshold"}, {"Level"=3, "Class Only"=TRUE, "Identifier"="", "Descriptive Name"="Decoding Results", "Data Type"=0, "Command"="", "Access"=0, "Range Table"="", "Read Callback"="", "Write Callback"="", "Supported Models"="", "Instrument Options"="", "Flags"=0, "Help"="Returns the decoding result of the specified packet."}, {"Level"=4, "Class Only"=FALSE, "Identifier"="RSSCOPE_ATTR_PROTOCOL_USB_DECODING_RESULTS_PACKET_COUNT", "Descriptive Name"="Protocol USB Decoding Results Packet Count", "Data Type"=0, "Command"="BUS{SerialBus}:USB:PCO?", "Access"=0, "Range Table"="", "Read Callback"="", "Write Callback"="", "Supported Models"="", "Instrument Options"="K60", "Flags"=0, "Help"="Returns the packet count for the selected serial bus, i.e. the number of packets in the present acquisition.\n\nAvailable Repeated Capabilities:\nSerialBus: SB1, SB2, SB3, SB4\r\n\nRemote-control command(s):\nBUS<m>:USB:PCOunt?"}, {"Level"=2, "Class Only"=TRUE, "Identifier"="", "Descriptive Name"="USB 31 Generation 1", "Data Type"=0, "Command"="", "Access"=0, "Range Table"="", "Read Callback"="", "Write Callback"="", "Supported Models"="", "Instrument Options"="", "Flags"=0, "Help"="R&S RTO-K61 is a firmware option that enables the R&S RTO to analyze Universal Serial Bus (USB) signals encoded by the USB 3.1 coding standard, generation 1."}, {"Level"=3, "Class Only"=FALSE, "Identifier"="RSSCOPE_ATTR_PROTOCOL_USB31_GEN1_SOURCE", "Descriptive Name"="Protocol USB31 Gen1 Source", "Data Type"=0, "Command"="BUS{SerialBus}:USBT:SOUR", "Access"=2, "Range Table"="rsscope_rngUSB31Gen1Source", "Read Callback"="", "Write Callback"="", "Supported Models"="", "Instrument Options"="K61", "Flags"=0, "Help"="Selects the source for the data signal in the USB 3.1 protocol.\n\nAvailable Repeated Capabilities:\nSerialBus: SB1, SB2, SB3, SB4\r\n\nRemote-control command(s):\nBUS<m>:USBThree:SOURce"}, {"Level"=3, "Class Only"=FALSE, "Identifier"="RSSCOPE_ATTR_PROTOCOL_USB31_GEN1_POLARITY", "Descriptive Name"="Protocol USB31 Gen1 Polarity", "Data Type"=0, "Command"="BUS{SerialBus}:USBT:POL", "Access"=2, "Range Table"="rsscope_rngUSB31Gen1Polarity", "Read Callback"="", "Write Callback"="", "Supported Models"="", "Instrument Options"="K61", "Flags"=0, "Help"="Defines the polarity of the data signal for the active (U0) state of the port.\n\nAvailable Repeated Capabilities:\nSerialBus: SB1, SB2, SB3, SB4\r\n\nRemote-control command(s):\nBUS<m>:USBThree:POLarity"}, {"Level"=3, "Class Only"=FALSE, "Identifier"="RSSCOPE_ATTR_PROTOCOL_USB31_GEN1_THRESHOLD_LOW", "Descriptive Name"="Protocol USB31 Gen1 Threshold Low", "Data Type"=1, "Command"="BUS{SerialBus}:USBT:THRL", "Access"=2, "Range Table"="RsScope_rngUSB31Gen1Threshold", "Read Callback"="", "Write Callback"="", "Supported Models"="", "Instrument Options"="K61", "Flags"=0, "Help"="Defines the lower threshold level for digitization of the data signal in the USB 3.1 protocol.\n\nAvailable Repeated Capabilities:\nSerialBus: SB1, SB2, SB3, SB4\r\n\nRemote-control command(s):\nBUS<m>:USBThree:THRLow"}, {"Level"=3, "Class Only"=FALSE, "Identifier"="RSSCOPE_ATTR_PROTOCOL_USB31_GEN1_THRESHOLD_HIGH", "Descriptive Name"="Protocol USB31 Gen1 Threshold High", "Data Type"=1, "Command"="BUS{SerialBus}:USBT:THRH", "Access"=2, "Range Table"="RsScope_rngUSB31Gen1Threshold", "Read Callback"="", "Write Callback"="", "Supported Models"="", "Instrument Options"="K61", "Flags"=0, "Help"="Defines the upper threshold level for digitization 
